vi "ConfigureUnits.vi"(4 "error in (no error)":errorcluster, 5 "velocity units":T1={"velocity dimension"=164, "velocity notation"=0} {"velocity notation" items=["standard"=0, "deci"=-1, "centi"=-2, "milli"=-3]; "velocity dimension" items=["revolution / time (rev/min)"=164]}, 7 "axis in":cluster{"keyHandle":u32, "nodeId":u16}={"keyHandle"=0, "nodeId"=1}) -> (0 "error out":errorcluster, 3 "axis out":cluster{"keyHandle":u32, "nodeId":u16}={"keyHandle"=0, "nodeId"=1})   [LabVIEW 2018]
doc: "<B>ConfigureUnits</B> writes the unit parameters for velocity to the device."
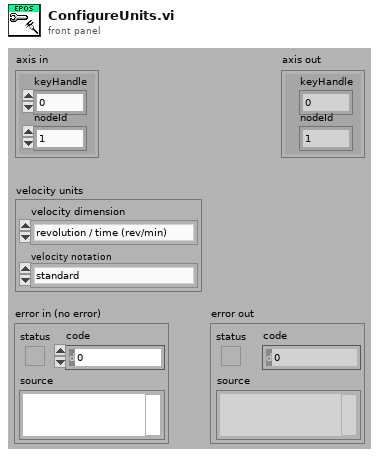
[diagram p1: front panel]
types:
  T1 = cluster{"velocity dimension":u8, "velocity notation":i8}
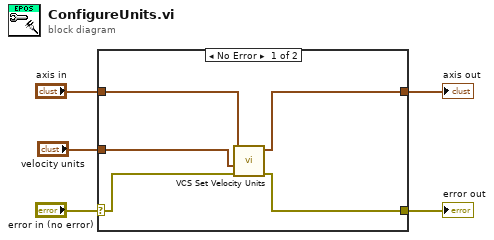
[diagram p0: block diagram]
diagram:
  n1 = case shown="No Error" "error in (no error)" {
    selector: "error in (no error)" -> [w10 w12]
    tunnel: [w9 w12] -> w4
    tunnel: [w8 w11] -> w3
    tunnel: "axis in" -> [w6 w11]
    tunnel: "velocity units" -> [w7 _]
    frame No Error {
      n2 = call "VCS Set Velocity Units.vi"("error in (no error)"=w10, "index"=w7, "axis in"=w6) -> ("error out"=w9:errorcluster, "axis out"=w8:cluster{"keyHandle":u32, "nodeId":u16})  [unwired: 7 in]
    }
    frame Error {
    }
  }
  "error out" <- w4
  "axis out" <- w3
